vi "pp2_sessList_createPseudoGellerman.vi"(8 "error in (no error)":errorcluster, 9 "Start Num":i32=2 min=0, 10 "Total Trials":i32=15 min=3 step=1, 11 "Trial Types":T1[](array[typedef])=[{"Trial Type Number"=1, "Trial Type"=enum."GO", "Trial Weight"=1, "Shock (mA)"=-1.0, "Duration (ms)"=250.0, "Sound Type"=enum."04 FM Sweep", "Stim P1"=2000.0, "Stim P2"=4000.0, "Stim P3"=0.0, "Stim P4"=0.0}, {"Trial Type Number"=2, "Trial Type"=enum."NOGO", "Trial Weight"=1, "Shock (mA)"=-1.0, "Duration (ms)"=250.0, "Sound Type"=enum."04 FM Sweep", "Stim P1"=4000.0, "Stim P2"=2000.0, "Stim P3"=0.0, "Stim P4"=0.0}] {"Shock (mA)" min=-1.0 max=5.0; "Trial Weight" step=1; "Duration (ms)" min=0.0 max=1.0; "Trial Type Number" min=1 step=1}) -> (0 "error out":errorcluster, 3 "Session List (Cannot Edit)":i32[](array[numeric]))   [LabVIEW 2013]
uses:
  pp2_Trial.ctl
  pp2_CTL_TrialType.ctl
  labolabo2/waveforms/WFTypes.ctl
  labolabo2/array/impl/NullArray_I.vi
  labolabo2/random/impl/RandomizeArray_I.vi
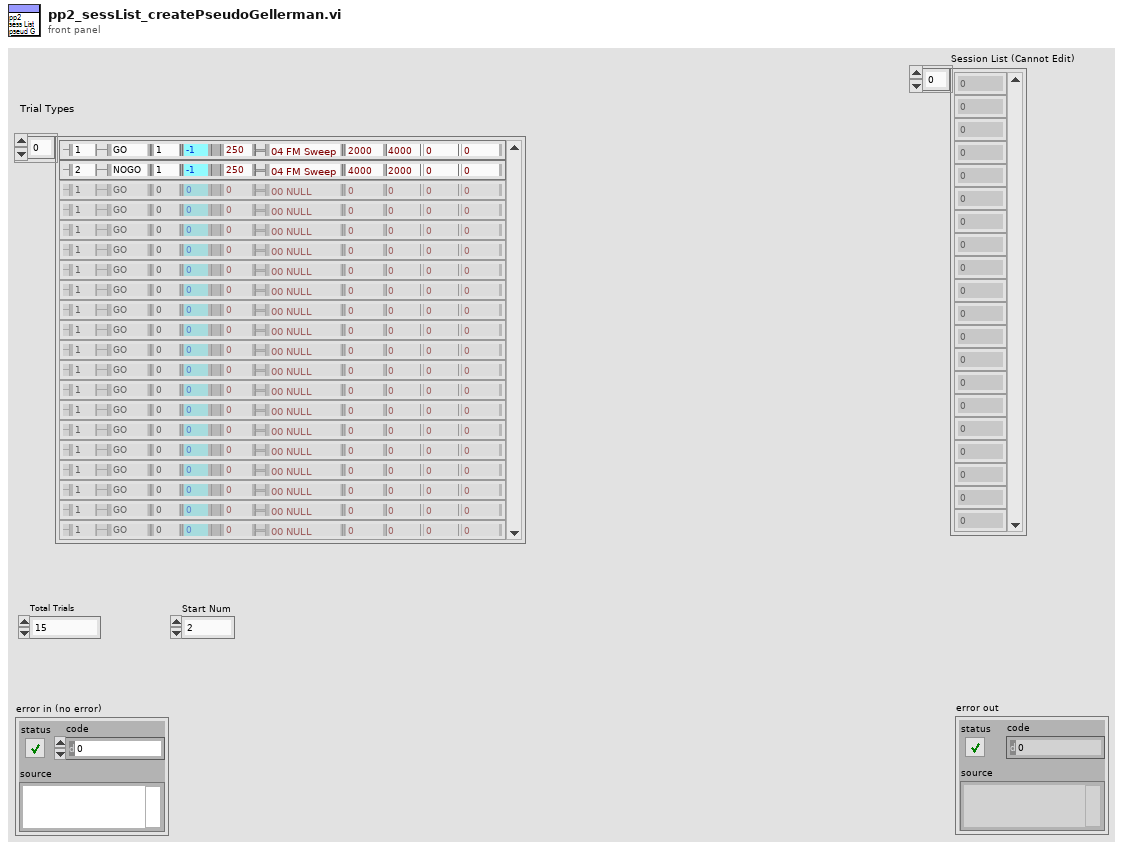
[diagram p1: front panel]
types:
  T1 = typedef "pp2_Trial.ctl" = cluster{"Trial Type Number":u8, "Trial Type":T2, "Trial Weight":u32, "Shock (mA)":dbl, "Duration (ms)":dbl, "Sound Type":T3, "Stim P1":dbl, "Stim P2":dbl, "Stim P3":dbl, "Stim P4":dbl}
  T2 = typedef "pp2_CTL_TrialType.ctl" = enum16{"OFF", "GO", "NOGO", "TEST"}
  T3 = typedef "WFTypes.ctl" = enum16{"00 NULL", "01 DC", "02 Noise", "03 Pure Tone", "04 FM Sweep"}
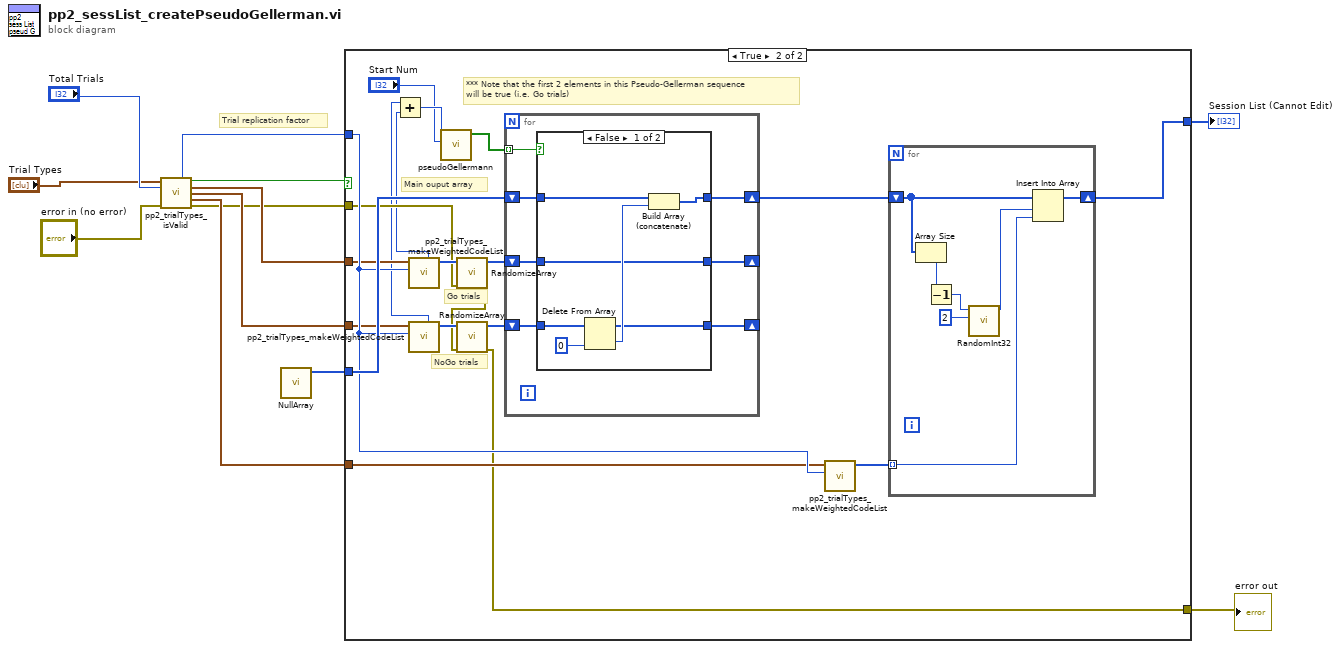
[diagram p0: block diagram]
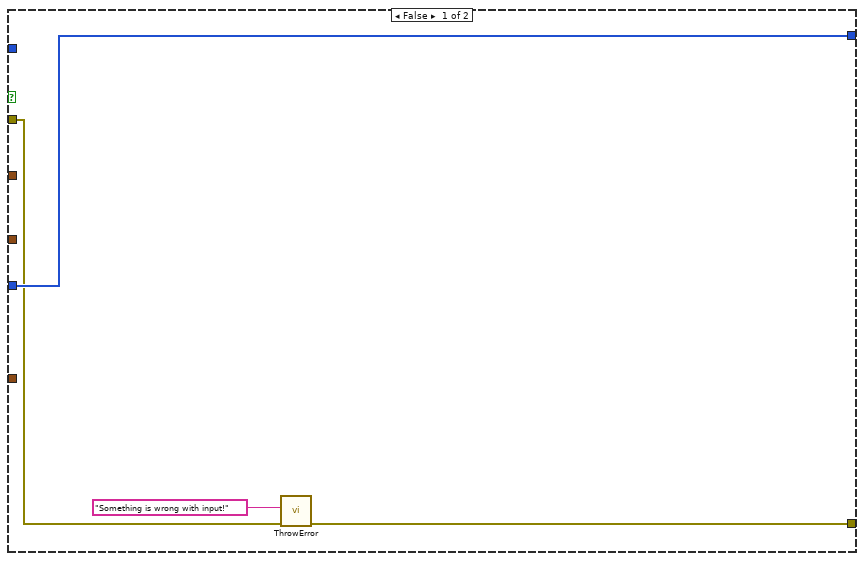
[diagram p2: hidden frame]
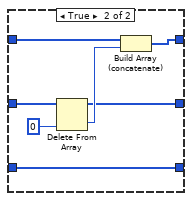
[diagram p3: hidden frame]
diagram:
  # "Trial replication factor"
  n1 = call "pp2_trialTypes_isValid.vi"("Trial Types In"="Trial Types", "Total Trials"="Total Trials", "error in (no error)"="error in (no error)") -> ("Trial Replication Factor"=w8:i32, "Paradigm Valid?"=w6:bool, "GO Trials"=w5:T1[], "NOGO Trials"=w4:T1[], "TEST Trials"=w3:T1[], "error out"=w2:errorcluster)  [unwired: 7 in]
  n2 = call-poly "NullArray.vi"() -> ("Null Array"=w12:i32[])  [unwired: 11 in]
  n3 = case shown="True" w6 {
    tunnel: w8 -> [_ w28]
    tunnel: w12 -> [w16 w31]
    tunnel: [w16 w29] -> w11
    tunnel: [w14 w22] -> w10
    tunnel: w5 -> [_ w27]
    tunnel: w4 -> [_ w26]
    tunnel: w3 -> [_ w25]
    tunnel: w2 -> [w13 w24]
    frame False {
      n4 = call "ThrowError.vi"("error in (no error)"=w13, "Error Message"="Something is wrong with input!" ("error message (\"\")")) -> ("error out"=w14:errorcluster)  [unwired: 8 in, 1 out]
    }
    frame True {
      # "*** Note that the first 2 elements in this Pseudo-Gellerman sequence\nwill be true (i.e. Go trials)"
      # "NoGo trials"
      # "Go trials"
      # "Main ouput array"
      n5 = call "pp2_trialTypes_makeWeightedCodeList.vi"("Trial Replication Factor"=w28, "Trial Types"=w27) -> ("Weighted Code List"=w34:i32[], "Weighted Code List Length"=w19:i32)  [unwired: 8 in]
      n6 = call "pp2_trialTypes_makeWeightedCodeList.vi"("Trial Replication Factor"=w28, "Trial Types"=w26) -> ("Weighted Code List"=w33:i32[], "Weighted Code List Length"=w18:i32)  [unwired: 8 in]
      n7 = Add(x=w18, y=w19) -> (x+y=w20:i32)
      n8 = call "pseudoGellermann.vi"("Start trues"="Start Num", "N"=w20) -> ("Array"=w36:bool[])  [unwired: 9 in]
      n9 = call-poly "RandomizeArray.vi"("error in (no error)"=w24, "Array In"=w34) -> ("error out"=w23:errorcluster, "Array Out"=w35:i32[])  [unwired: 8 in]
      n10 = call-poly "RandomizeArray.vi"("error in (no error)"=w23, "Array In"=w33) -> ("error out"=w22:errorcluster, "Array Out"=w32:i32[])  [unwired: 8 in]
      n11 = for {
        tunnel: w36 -> [w50] mode=indexing
        shift-right: [w45] -> _
        shift-left: w35 -> [w46]
        shift-right: [w47] -> _
        shift-left: w32 -> [w48]
        shift-right: [w44] -> w30
        shift-left: w31 -> [w49]
        n12 = case shown="False" w50 {
          tunnel: [w56 w63] -> w44
          tunnel: w49 -> [w55 w62]
          tunnel: w48 -> [w53 w61]
          tunnel: [w52 w61] -> w47
          tunnel: w46 -> [w51 w60]
          tunnel: [w51 w58] -> w45
          frame False {
            n13 = Delete From Array(array=w53, index=0 ("index (row)")) -> (deleted portion=w54:i32, array with subset deleted=w52:i32[])  [unwired: 1 in]
            n14 = Build Array (concatenate)(w55, w54) -> (w56:i32[])
          }
          frame True {
            n15 = Delete From Array(array=w60, index=0 ("index (row)")) -> (deleted portion=w59:i32, array with subset deleted=w58:i32[])  [unwired: 1 in]
            n16 = Build Array (concatenate)(w62, w59) -> (w63:i32[])
          }
        }
      }
      n17 = call "pp2_trialTypes_makeWeightedCodeList.vi"("Trial Replication Factor"=w28, "Trial Types"=w25) -> ("Weighted Code List"=w21:i32[])  [unwired: 8 in, 1 out]
      n18 = for {
        tunnel: w21 -> [w38] mode=indexing
        shift-right: [w39] -> w29
        shift-left: w30 -> [w40]
        n19 = Array Size(array=w40) -> (size(s)=w41:i32)
        n20 = Decrement(x=w41) -> (x-1=w42:i32)
        n21 = call "RandomInt32.vi"("Min"=2, "Max"=w42) -> ("Random"=w37:i32)  [unwired: 9 in]
        n22 = Insert Into Array(array=w40, index=w37, new element=w38) -> (w39:i32[])
      }
    }
  }
  "error out" <- w10
  "Session List (Cannot Edit)" <- w11
